vi "Read Breakpoint.vi"(8 "error in (no error)":errorcluster, 11 "abs_Node in":refnum<class "abs_Node.lvclass">) -> (0 "error out":errorcluster, 2 "Breakpoint":bool, 3 "abs_Node out":refnum<class "abs_Node.lvclass">)   [LabVIEW 2021, in "BT.lvlib" / "abs_Node.lvclass"]
uses:
  abs_Node.lvclass
  abs_Node.lvclass/abs_Node.ctl
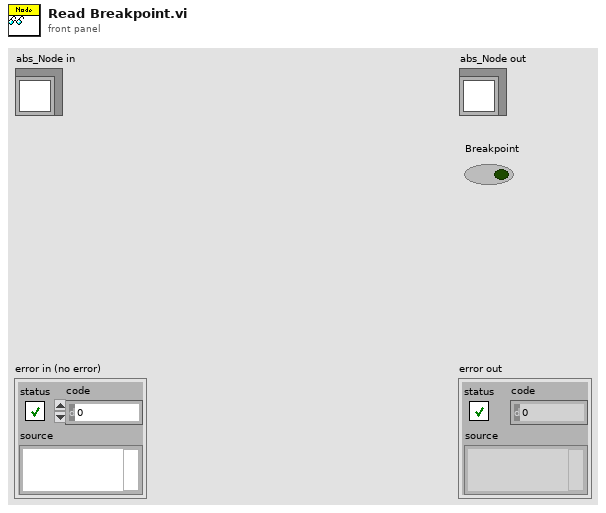
[diagram p1: front panel]
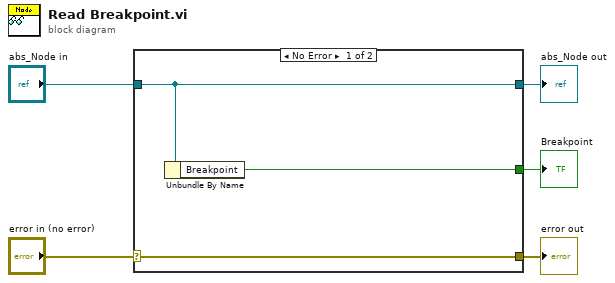
[diagram p0: block diagram]
diagram:
  n1 = case shown="No Error" "error in (no error)" {
    selector: "error in (no error)" -> [w8 w9]
    tunnel: [w8 w9] -> w4
    tunnel: [w7 w10] -> w2
    tunnel: "abs_Node in" -> [w7 w10]
    tunnel: [w6 _] -> w1
    frame No Error {
      n2 = Unbundle By Name(w7) -> ("Breakpoint"=w6:bool)
    }
    frame Error {
    }
  }
  "error out" <- w4
  "abs_Node out" <- w2
  "Breakpoint" <- w1
